vi "Porcentaje_Delta.vi"(3 "Array in":dbl[](array[numeric])) -> (0 "Array":dbl[](array[numeric]), 1 "Numeric Control":i32)   [LabVIEW 2017]
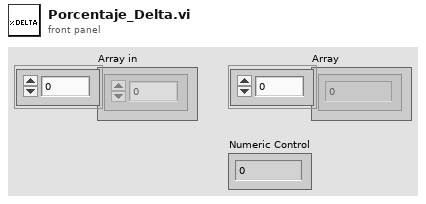
[diagram p1: front panel]
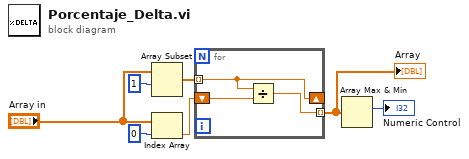
[diagram p0: block diagram]
diagram:
  n1 = Array Subset(array="Array in", index=1) -> (w6:dbl[])  [unwired: 1 in]
  n2 = Index Array(array="Array in", index=0) -> (element=w4:dbl)
  n3 = for {
    tunnel: [w9] -> w1 mode=indexing
    shift-right: [w8] -> _
    shift-left: w4 -> [w10]
    tunnel: w6 -> [w8] mode=indexing
    n4 = Divide(x=w8, y=w10) -> (x/y=w9:dbl)
  }
  "Array" <- w1
  n5 = Array Max & Min(array=w1) -> (max index (indices)=→"Numeric Control":i32)  [unwired: 3 out]
